vi "CRYCCITT_LR.vi"(0 "Weight [Hz,dB]":cluster{dbl, dbl}[](array[cluster])=[{100.0, 154.0}, {125.0, 115.4}, {160.0, 89.0}, {200.0, 77.2}, {315.0, 62.3}, {400.0, 45.0}, {500.0, 53.4}, {630.0, 48.8}, {800.0, 47.9}, {1000.0, 50.4}, {1250.0, 59.4}, {1600.0, 57.0}, {2000.0, 72.5}, {2500.0, 72.9}, {3150.0, 89.5}, {4000.0, 117.3}, {5000.0, 157.3}, {6300.0, 172.2}, {8000.0, 181.7}] {"?" format="%.2f"; "?" format="%.2f"}, 2 "Freq. Response [Hz,dB]":cluster{dbl, dbl}[](array[cluster])=[{100.0, 4.334660686771568}, {106.0, 5.373350538440173}, {112.0, 6.355548973814951}, {118.0, 7.300104104118085}, {125.0, 8.337607175181217}, {132.0, 9.331226001934875}, {140.0, 10.437014672651827}, {150.0, 11.730182148662191}, {160.0, 12.944269069963623}, {170.0, 14.081999072641498}, {180.0, 15.154678812807605}, {190.0, 16.167710416411012}, {200.0, 16.69901938888695}, {212.0, 17.943101442819255}, {224.0, 18.80012659830309}, {236.0, 19.5334215651581}, {250.0, 20.219127511607763}, {265.0, 20.801317746415418}, {280.0, 21.229152829510408}, {300.0, 21.605015780679633}, {315.0, 21.773212893618382}, {335.0, 21.804667075972386}, {355.0, 21.837198881991657}, {375.0, 21.485523479208762}, {400.0, 22.213959843111738}, {425.0, 22.00674187976686}, {450.0, 21.81955771330965}, {475.0, 21.70978945691449}, {500.0, 21.631496018393385}, {530.0, 21.525639840927123}, {560.0, 21.476205594993413}, {600.0, 21.43884029107397}, {630.0, 21.42981717122098}, {670.0, 21.41033857955144}, {710.0, 21.352551022383295}, {750.0, 21.39271774796619}, {800.0, 21.44836325921421}, {850.0, 21.56048529643944}, {900.0, 21.763051724631577}, {950.0, 22.061559763299506}, {1000.0, 22.35574541921071}, {1060.0, 22.609816250143915}, {1120.0, 22.98516747163893}, {1180.0, 23.389352951246302}, {1250.0, 23.791554974887752}, {1320.0, 24.1331425727989}, {1400.0, 24.432535228090426}, {1500.0, 24.59039005448819}, {1600.0, 24.359604688072505}, {1700.0, 24.028623866959265}, {1800.0, 23.559905387723163}, {1900.0, 23.185525970868195}, {2000.0, 22.814584972330184}, {2120.0, 22.785596118616414}, {2240.0, 22.905192973907997}, {2360.0, 23.031480048076496}, {2500.0, 23.26863455994114}, {2650.0, 23.82717255847565}, {2800.0, 24.140307857563727}, {3000.0, 24.166210358118146}, {3150.0, 24.042333935789987}, {3350.0, 23.533534605486203}, {3550.0, 22.89485448945683}, {3750.0, 22.47259355936781}, {4000.0, 22.416201171782845}, {4250.0, 22.02481274774421}, {4500.0, 18.185500243742176}, {4750.0, 11.424847264673964}, {5000.0, 6.421554604417297}, {5300.0, 2.4508959525975498}, {5600.0, 0.09594649440220801}, {6000.0, -1.3792335657355383}, {6300.0, -2.472373893894961}, {6700.0, -3.0915543461988504}, {7100.0, -3.976722203641198}, {7500.0, -5.11436396211375}, {8000.0, -6.294315220489285}, {8500.0, -7.635013072331965}, {9000.0, -2.217987481522152}, {9500.0, 2.850712516650384}, {10000.0, 2.8682236396937233}] {"?" format="%.2f"; "?" format="%.2f"}, 3 "Exponent":dbl=0.175 format="%.3f", 4 "dB Correction [dB]":dbl format="%.2f") -> (5 "LR [dB]":dbl=0.021631825077412792 format="%.2f")   [LabVIEW 2013]
panel:
  # "This VI calculates the CCITT Rec. P79 Loudness Rating from the values in Freq.Response.\n\nThe formula is:\n\n LR = -(10/Exponent)*Log10( Sum( 10 raised to( (Freq.Resp - Weight)*Exponent/10 ) ) )\n\ndB Correction is added to Freq. Response, and may be used to correct for different dB references (e.g. if Freq. Response is dB rel 1 mV/Pa and the LR shall be dB rel 1 V/Pa, the dB Correction shall be -60 dB).\n\nThe VI can use any Freq. Response with at least one point."
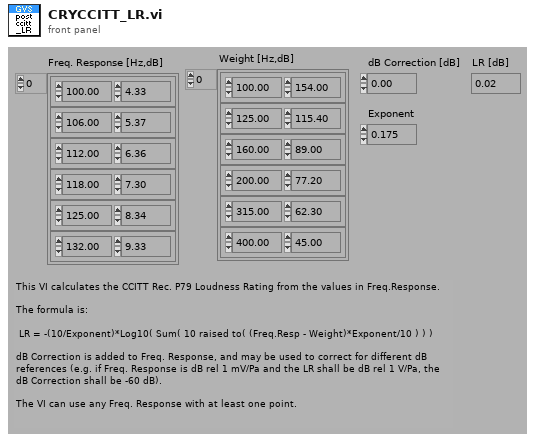
[diagram p1: front panel]
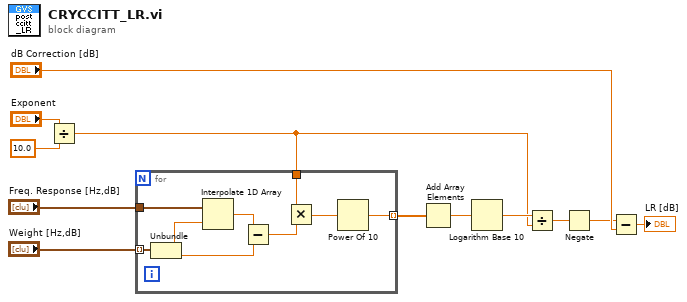
[diagram p0: block diagram]
diagram:
  n1 = Divide(x="Exponent", y=10.0) -> (x/y=w1:dbl)
  n2 = for {
    tunnel: "Weight [Hz,dB]" -> [w21] mode=indexing
    tunnel: "Freq. Response [Hz,dB]" -> [w13]
    tunnel: w1 -> [w17]
    tunnel: [w14] -> w6 mode=indexing
    n3 = Unbundle(w21) -> (w19:dbl, w18:dbl)
    n4 = Interpolate 1D Array(1:w19, 2:w13) -> (0:w20:dbl)
    n5 = Subtract(x=w20, y=w18) -> (x-y=w16:dbl)
    n6 = Multiply(x=w17, y=w16) -> (x*y=w15:dbl)
    n7 = Power Of 10(x=w15) -> (10^x=w14:dbl)
  }
  n8 = Add Array Elements(numeric array=w6) -> (sum=w5:dbl)
  n9 = Logarithm Base 10(1:w5) -> (0:w2:dbl)
  n10 = Divide(x=w2, y=w1) -> (x/y=w4:dbl)
  n11 = Negate(x=w4) -> (-x=w3:dbl)
  n12 = Subtract(x=w3, y="dB Correction [dB]") -> (x-y=→"LR [dB]":dbl)
